vi "analyze data.vi"(9 "Graph array":cluster{"output":dbl[], "output":dbl[]}[](array[cluster]), 10 "Y-columns":dbl[](array[numeric]), 11 "selected files2":T2(array[cluster])) -> ()   [LabVIEW 2020]
panel:
  in  "(5) analysis":T1(ring)
  out "concatenated string":string
  in  "(6) Done":bool
  in  "(3) use custom \nvariables?":bool
  in  "(4) variables\n (should be filled)":string
  in  "file path (dialog if empty)":path
  in  "(2) Y-column names":string[](array[string])
  in  "(1) x-axis title":string
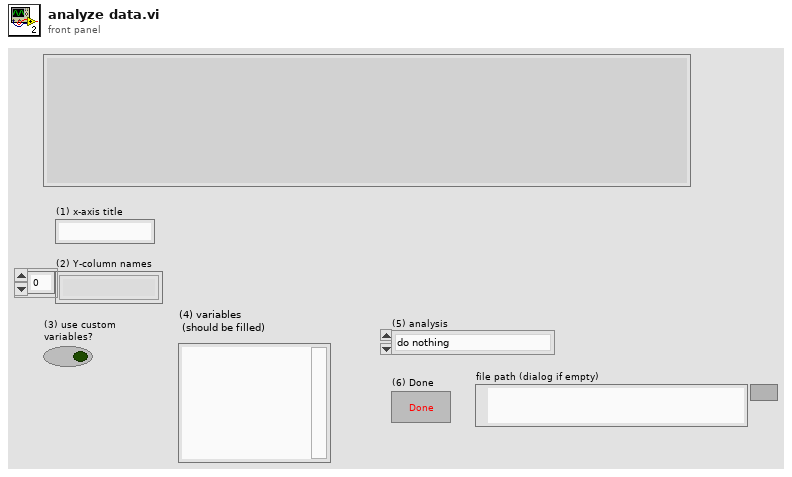
[diagram p1: front panel]
types:
  T1 = enum16{"do nothing", "FFT", "Relaxation", "Non-linear curve fit", "Simple math and reader", "MR analysis", "Thermal K data"}
  T2 = cluster{"String":string, "Boolean":bool, "begin":u32, "length":u32, "Numeric":dbl}[]
  T3 = enum16{"do nothing", "FFT", "Relaxation", "Non-linear curve fit", "Simple math and reader"}
  T4 = enum16{"Save as Ascill file", "write to clipboard", "do not export"}
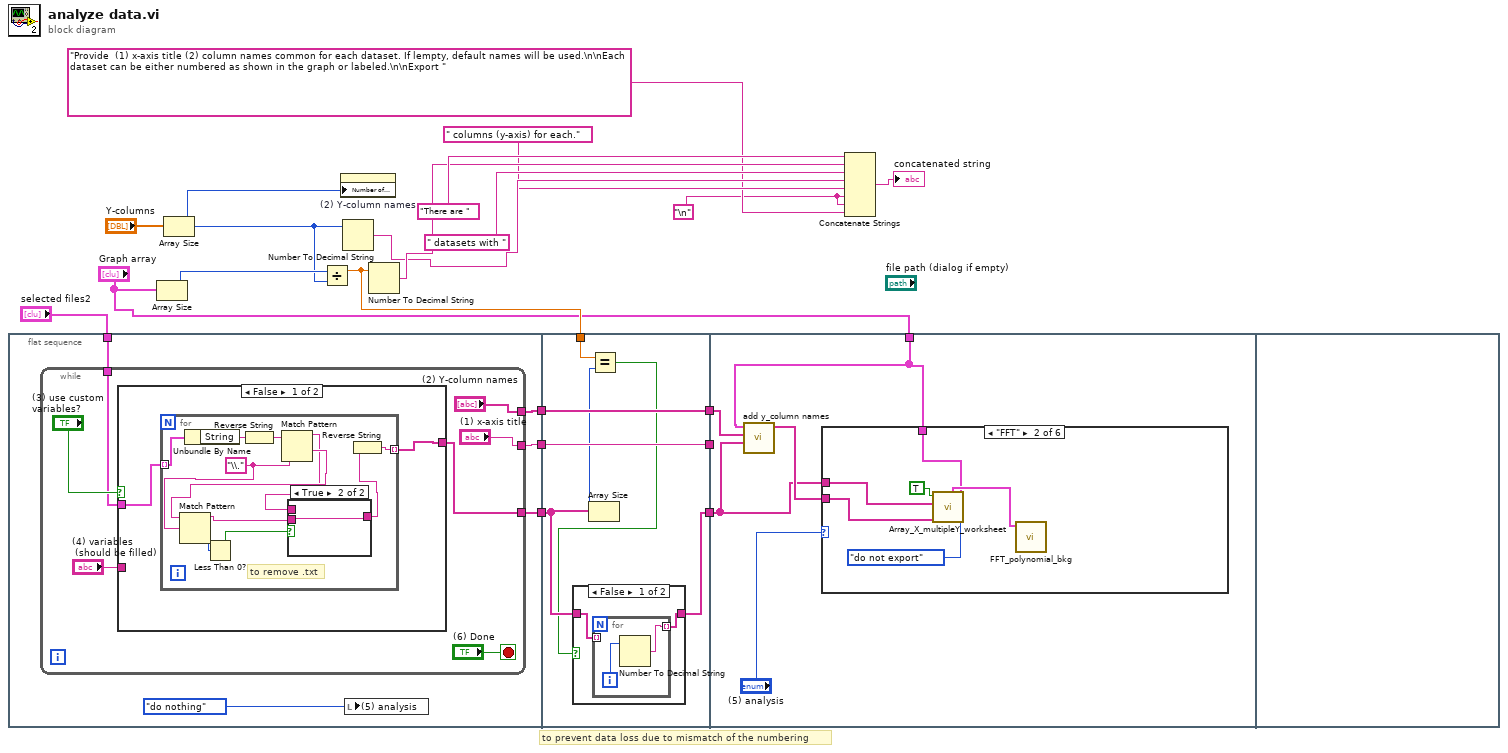
[diagram p0: block diagram]
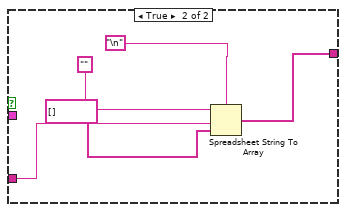
[diagram p3: hidden frame]
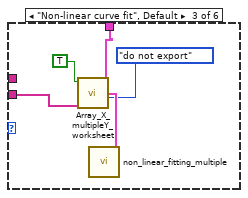
[diagram p6: hidden frame]
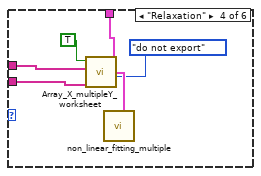
[diagram p7: hidden frame]
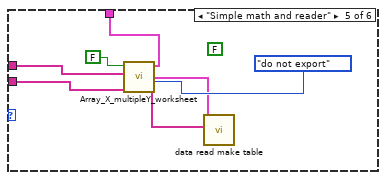
[diagram p8: hidden frame]
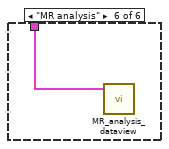
[diagram p9: hidden frame]
diagram:
  w9 = "\n"
  # "to prevent data loss due to mismatch of the numbering"
  n1 = flat-sequence {
    tunnel: [w25] -> w8
    tunnel: [w24] -> w6
    tunnel: [w23] -> w4
    tunnel: "selected files2" -> [w22]
    tunnel: w8 -> [w59]
    tunnel: [w59] -> w7
    tunnel: w6 -> [w58]
    tunnel: [w58] -> w5
    tunnel: w4 -> [w55]
    tunnel: w3 -> [w56]
    tunnel: [w54] -> w2
    tunnel: w7 -> [w68]
    tunnel: w5 -> [_]
    tunnel: w2 -> [w66]
    tunnel: "Graph array" -> [w69]
    frame #0 {
      n2 = while {
        tunnel: ["(2) Y-column names"] -> w25
        tunnel: ["(1) x-axis title"] -> w24
        tunnel: [w29] -> w23
        tunnel: w22 -> [w27]
        stop <- "(6) Done" stop-if-true
        n3 = case shown="False" "(3) use custom \nvariables?" {
          tunnel: [w33 w49] -> w29
          tunnel: w27 -> [w34 _]
          tunnel: "(4) variables\n (should be filled)" -> [_ w48]
          frame False {
            n4 = for {
              tunnel: [w43] -> w33 mode=indexing
              tunnel: w34 -> [w42] mode=indexing
              w41 = "\\." ("regular expression")
              # "to remove .txt"
              n5 = Unbundle By Name(w42) -> ("String"=w45:string)
              n6 = Reverse String(1:w45) -> (0:w44:string)
              n7 = Match Pattern(string=w44, regular expression=w41) -> (before substring=w35:string, after substring=w36:string)  [unwired: 1 in, 2 out]
              n8 = Match Pattern(string=w36, regular expression=w41) -> (before substring=w37:string, offset past match=w39:i32)  [unwired: 1 in, 2 out]
              n9 = Less Than 0?(x=w39) -> (x < 0?=w38:bool)
              n10 = case shown="True" w38 {
                tunnel: w35 -> [_ w47]
                tunnel: [w46 w47] -> w40
                tunnel: w37 -> [w46 _]
                frame False {
                }
                frame True {
                }
              }
              n11 = Reverse String(1:w40) -> (0:w43:string)
            }
          }
          frame True {
            n12 = Spreadsheet String To Array(delimiter (Tab)="\n", format string="", spreadsheet string=w48, array type (2D Dbl)=string[] []) -> (array=w49:string[])
          }
        }
      }
      n13 = local write "(5) analysis"(T3."do nothing" ("(5) analysis")) -> ()
    }
    frame #1 {
      n14 = Array Size(array=w55) -> (size(s)=w57:i32)
      n15 = Equal?(x=w56, y=w57) -> (x = y?=w53:bool)
      n16 = case shown="False" w53 {
        tunnel: w55 -> [w61 w64]
        tunnel: [w60 w64] -> w54
        frame False {
          n17 = for {
            tunnel: w61 -> [_] mode=indexing
            tunnel: [w62] -> w60 mode=indexing
            i -> [w63]
            n18 = Number To Decimal String(number=w63) -> (decimal integer string=w62:string)  [unwired: 1 in]
          }
        }
        frame True {
        }
      }
    }
    frame #2 {
      n19 = call "add y_column names.vi"("column extension"=w66, "old y-column names"=w68, "graph file"=w69) -> ("new y-column names"=w67:string[])  [unwired: 6 in, 2 out]
      n20 = case shown="\"FFT\"" "(5) analysis" {
        tunnel: w66 -> [_ w72 _ w82 w89 _]
        tunnel: w67 -> [_ w71 w78 w84 w88 _]
        tunnel: w69 -> [_ w70 w77 w83 w90 w94]
        frame "do nothing" {
        }
        frame "FFT" {
          n21 = call "Array_X_multipleY_worksheet.vi"("Sort?"=TRUE, "column extension"=w72, "Y-column names"=w71, "graph file"=w70, "export"=T4."do not export") -> ("Graph array"=w73:cluster{"output":dbl[], "output":dbl[]}[])  [unwired: 2 in, 1 out]
          n22 = call "FFT_polynomial_bkg.vi"("Graph array"=w73) -> ()  [unwired: 11 in]
        }
        frame "Non-linear curve fit", Default {
          n23 = call "Array_X_multipleY_worksheet.vi"("Sort?"=TRUE, "Y-column names"=w78, "graph file"=w77, "export"=T4."do not export") -> ("Graph array"=w79:cluster{"output":dbl[], "output":dbl[]}[])  [unwired: 3 in, 1 out]
          n24 = call "non_linear_fitting_multiple.vi"("Graph array"=w79) -> ()  [unwired: 10 in, 1 out]
        }
        frame "Relaxation" {
          n25 = call "Array_X_multipleY_worksheet.vi"("Sort?"=TRUE, "column extension"=w82, "Y-column names"=w84, "graph file"=w83, "export"=T4."do not export") -> ("Graph array"=w85:cluster{"output":dbl[], "output":dbl[]}[])  [unwired: 2 in, 1 out]
          n26 = call "non_linear_fitting_multiple.vi"("Graph array"=w85) -> ()  [unwired: 10 in, 1 out]
        }
        frame "Simple math and reader" {
          (unwired) FALSE ("save ascii")
          n27 = call "Array_X_multipleY_worksheet.vi"("Sort?"=FALSE, "column extension"=w89, "Y-column names"=w88, "graph file"=w90, "export"=T4."do not export") -> ("Graph array"=w91:cluster{"output":dbl[], "output":dbl[]}[], "new y-column names"=w87:string[])  [unwired: 2 in]
          n28 = call "data read make table.vi"("new y-column names"=w87, "Graph array"=w91) -> ()  [unwired: 10 in]
        }
        frame "MR analysis" {
          n29 = call "MR_analysis_dataview.vi"("Raw data Y(X) at different Z"=w94) -> ()  [unwired: 5 in]
        }
      }
    }
    frame #3 {
    }
  }
  n30 = Array Size(array="Graph array") -> (size(s)=w18:i32)
  n31 = Array Size(array="Y-columns") -> (size(s)=w14:i32)
  n32 = Divide(x=w18, y=w14) -> (x/y=w3:dbl)
  n33 = property on="(2) Y-column names" class="Arr (strict)"("Number of Columns"=w14) -> ()  [unwired: 2 in, 2 out]
  n34 = Number To Decimal String(number=w14) -> (decimal integer string=w13:string)  [unwired: 1 in]
  n35 = Number To Decimal String(number=w3) -> (decimal integer string=w16:string)  [unwired: 1 in]
  n36 = Concatenate Strings("There are ", w16, " datasets with " ("string"), w13, " columns (y-axis) for each." ("string"), w9, w9, "Provide  (1) x-axis title (2) column names common for each dataset. If lempty, default names will be used.\n\nEach dataset can be either numbered as shown in the graph or labeled.\n\nExport " ("string")) -> (→"concatenated string":string)
